vi "SetTableSelect.vi"(6 "キー列(0)":i32, 8 "error in (no error)":errorcluster caption="エラー入力（エラーなし）", 9 "強制NORMAL(f)":bool, 10 "選択文字":string, 11 "Table ref":refnum<vi>) -> (0 "error out":errorcluster caption="エラー出力", 2 "選択文字(copy)":string, 3 "Table ref (copy)":refnum<vi>)   [LabVIEW 2014]
uses:
  <vilib>/Utility/miscctls.llb/LVRowAndColumnTypeDef.ctl
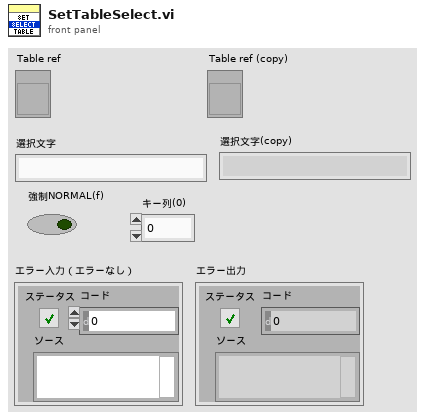
[diagram p1: front panel]
types:
  T1 = typedef "LVRowAndColumnTypeDef.ctl" = cluster{"Row":i32, "Column":i32}
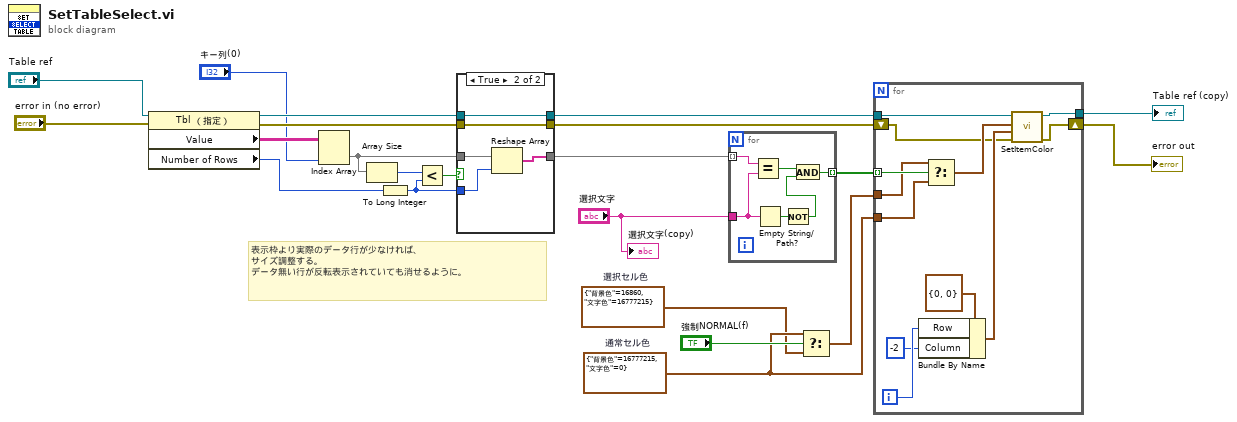
[diagram p0: block diagram]
diagram:
  w15 = cluster{"背景色":u32, "文字色":u32} {"背景色"=16860, "文字色"=16777215}  # 選択セル色
  w16 = cluster{"背景色":u32, "文字色":u32} {"背景色"=16777215, "文字色"=0}  # 通常セル色
  # "表示枠より実際のデータ行が少なければ、\nサイズ調整する。\nデータ無い行が反転表示されていても消せるように。"
  n1 = property class="Tbl （指定）"(reference="Table ref", error in="error in (no error)") -> (reference out=w2:refnum<vi>, error out=w4:errorcluster, "Value"=w22:string[][], "Number of Rows"=w8:u32)
  n2 = Index Array(array=w22, index (col)="キー列(0)") -> (element=w10:string[])  [unwired: 1 in]
  n3 = Array Size(array=w10) -> (size(s)=w9:i32)
  n4 = To Long Integer(number=w8) -> (32bit integer=w7:i32)
  n5 = Less?(x=w9, y=w7) -> (x < y?=w6:bool)
  n6 = case shown="TRUE" w6 {
    tunnel: [w23 w30] -> w12
    tunnel: w10 -> [w23 w29]
    tunnel: w7 -> [_ w28]
    tunnel: [w24 w27] -> w5
    tunnel: w4 -> [w24 w27]
    tunnel: [w25 w26] -> w3
    tunnel: w2 -> [w25 w26]
    frame False {
    }
    frame True {
      n7 = Reshape Array(w29, w28) -> (w30:string[])
    }
  }
  n8 = for {
    tunnel: w12 -> [w36] mode=indexing
    tunnel: "選択文字" -> [w35]
    tunnel: [w32] -> w20 mode=indexing
    n9 = Equal?(x=w36, y=w35) -> (x = y?=w33:bool)
    n10 = Empty String/Path?(string/path=w35) -> (empty?=w34:bool)
    n11 = Not(x=w34) -> (.not. x?=w31:bool)
    n12 = And(x=w33, y=w31) -> (x .and. y?=w32:bool)
  }
  n13 = Select(t=w16, s="強制NORMAL(f)", f=w15) -> (s? t:f=w14:cluster{"背景色":u32, "文字色":u32})
  n14 = for {
    tunnel: w20 -> [w45] mode=indexing
    tunnel: w14 -> [w44]
    tunnel: w16 -> [w43]
    tunnel: w3 -> [w41]
    shift-right: [w38] -> w19
    shift-left: w5 -> [w39]
    tunnel: [w37] -> w18
    i -> [w47]
    n15 = Bundle By Name(cluster=T1 {"Row"=0, "Column"=0} ("行列指定"), "Row"=w47, "Column"=-2) -> (w40:T1)
    n16 = Select(t=w44, s=w45, f=w43) -> (s? t:f=w42:cluster{"背景色":u32, "文字色":u32})
    n17 = call "SetItemColor.vi"("エラー入力(エラーなし)"=w39, "行列指定"=w40, "色指定"=w42, "Tbl refnum"=w41) -> ("エラー出力"=w38:errorcluster, "Tbl refnum出力"=w37:refnum<vi>)  [unwired: 6 in]
  }
  "error out" <- w19
  "Table ref (copy)" <- w18
  "選択文字(copy)" <- "選択文字"
